vi "PelletSize_SubVI.vi"(11 "BrickReference in":T1) -> (2 "Boolean":bool, 3 "BrickReference out":T1)   [LabVIEW 2016]
uses:
  <vilib>/NXT/Subs/LVHSConnector.ctl
  <vilib>/NXT/LegoClasses/BrickReference/BrickReference.lvclass
  <vilib>/NXT/Block Support/NXT_InputPort.ctl
  <vilib>/NXT/Dual Mode Library/Sensors/EV3_Ultrasonic_CM.vi
  <vilib>/NXT/NXTIO Xnodes/AddressXNode/NXTIOAddress.xnode
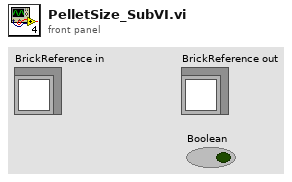
[diagram p1: front panel]
types:
  T1 = typedef "LVHSConnector.ctl" = refnum<class "BrickReference.lvclass">
  T2 = typedef "NXT_InputPort.ctl" = u32
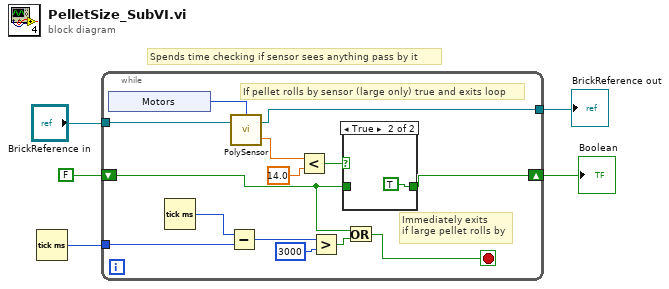
[diagram p0: block diagram]
diagram:
  # "Spends time checking if sensor sees anything pass by it"
  n1 = Tick Count (ms)() -> (millisecond timer value=w2:u32)
  n2 = while {
    shift-right: [w18] -> w4
    shift-left: FALSE -> [w7]
    tunnel: [w12] -> w1
    tunnel: w2 -> [w11]
    tunnel: "BrickReference in" -> [w9]
    stop <- w6 stop-if-true
    # "Immediately exits\nif large pellet rolls by"
    # "If pellet rolls by sensor (large only) true and exits loop"
    n3 = xnode "Motors"() -> ("Sensor"=w10:T2)
    n4 = Tick Count (ms)() -> (millisecond timer value=w16:u32)
    n5 = Subtract(x=w16, y=w11) -> (x-y=w15:u32)
    n6 = call-poly <vilib>:"PolySensor.vi"("NXT/EV3"=w9, "Port (Port 1)"=w10) -> ("Centimeters"=w13:sgl, "NXT/EV3"=w12:T1)  [unwired: 1 in]
    n7 = Less?(x=w13, y=sgl 14.0) -> (x < y?=w17:bool)
    n8 = Greater?(x=w15, y=u32 3000) -> (0:w8:bool)
    n9 = case shown="True" w17 {
      tunnel: w7 -> [w21 _]
      tunnel: [w21 TRUE] -> w18
      frame False {
      }
      frame True {
      }
    }
    n10 = Or(x=w7, y=w8) -> (x .or. y?=w6:bool)
  }
  "Boolean" <- w4
  "BrickReference out" <- w1
